vi "HFRR ADV v04 new software.vi"() -> ()   [LabVIEW 2025] (continued)
                n290 = Wait (ms)(milliseconds to wait=u32 1500) -> ()  [unwired: 1 out]
              }
            }
          }
        }
      }
      event "Headen Service Button": Value Change {
        n291 = event-data() -> ()  [unwired: 1 in, 6 out]
        n292 = local read "Headen Service Button"() -> (w388:bool)
        n293 = case shown="True" w388 {
          frame False {
            n294 = property on="Password 3" class="Clust (strict)"("Visible"=FALSE) -> ()  [unwired: 2 in, 2 out]
            n295 = property on="Service Password Log" class="Str"("Visible"=FALSE) -> ()  [unwired: 2 in, 2 out]
          }
          frame True {
            n296 = property on="Password 3" class="Clust (strict)"("Visible"=TRUE) -> ()  [unwired: 2 in, 2 out]
            n297 = property on="Service Password Log" class="Str"("Visible"=TRUE) -> ()  [unwired: 2 in, 2 out]
          }
        }
      }
      event "Password 3.Service Password": Value Change {
        n298 = event-data() -> ()  [unwired: 1 in, 6 out]
        n299 = Unbundle By Name("Password 3") -> ("Service Password"=w395:string)
        n300 = call <vilib>:"Trim Whitespace.vi"("string"=w395) -> ("trimmed string"=w393:string)  [unwired: 1 in]
        n301 = Equal?(x=w393, y="Service@123") -> (x = y?=w394:bool)
        n302 = case shown="False" w394 {
          selector: w394 -> [w399 w401]
          frame False {
            n303 = local write "Service Password enable"(w399) -> ()
            n304 = property on="Service Password Log" class="Str"("Visible"=TRUE) -> ()  [unwired: 2 in, 2 out]
            n305 = property on="Tab Control 5" class="TabCtl (strict)"("Tabs Visible?"=TRUE ("Page Labels Display Visible?")) -> ()  [unwired: 2 in, 2 out]
          }
          frame True {
            n306 = property on="Service Password Log" class="Str"("Visible"=FALSE) -> ()  [unwired: 2 in, 2 out]
            "Service Password enable" <- w401
          }
        }
      }
      event "Sign In": Value Change {
        w403 = FALSE ("Visible")
        n307 = event-data() -> ()  [unwired: 1 in, 6 out]
        n308 = property on="About" class="Clust (strict)"("Visible"=w403) -> ()  [unwired: 2 in, 2 out]
        n309 = property on="Password 3" class="Clust (strict)"("Visible"=w403) -> ()  [unwired: 2 in, 2 out]
        n310 = property on="Service Password Log" class="Str"("Visible"=FALSE) -> ()  [unwired: 2 in, 2 out]
      }
      event "Info": Value Change {
        n311 = event-data() -> ()  [unwired: 1 in, 6 out]
        n312 = local read "Info"() -> (w405:bool)
        n313 = case shown="False" w405 {
          frame False {
            n314 = property on="About" class="Clust (strict)"("Visible"=FALSE) -> ()  [unwired: 2 in, 2 out]
          }
          frame True {
            n315 = property on="About" class="Clust (strict)"("Visible"=TRUE) -> ()  [unwired: 2 in, 2 out]
          }
        }
      }
      event "Calibration": Value Change {
        n316 = event-data() -> ()  [unwired: 1 in, 6 out]
        n317 = local read "Calibration"() -> (w409:bool)
        n318 = case shown="False" w409 {
          frame False {
            n319 = property on="Calibration 2" class="TabCtl (strict)"("Visible"=FALSE) -> ()  [unwired: 2 in, 2 out]
            n320 = local write "Cal Password"("" ("Cal Password")) -> ()
          }
          frame True {
            n321 = property on="Calibration 2" class="TabCtl (strict)"("Visible"=TRUE) -> ()  [unwired: 2 in, 2 out]
            n322 = local write "Cal Password"("" ("Cal Password")) -> ()
          }
        }
        n323 = property on="Wrong Password" class="Str"("Visible"=FALSE) -> ()  [unwired: 2 in, 2 out]
      }
      event "Cal Password": Value Change {
        n324 = event-data() -> ()  [unwired: 1 in, 6 out]
        n325 = local read "Cal Password"() -> (w417:string)
        n326 = call <vilib>:"Trim Whitespace.vi"("string"=w417) -> ("trimmed string"=w416:string)  [unwired: 1 in]
        n327 = Equal?(x=w416, y="Cal@321") -> (x = y?=w414:bool)
        n328 = case shown="True" w414 {
          frame False {
            n329 = property on="Wrong Password" class="Str"("Visible"=TRUE) -> ()  [unwired: 2 in, 2 out]
          }
          frame True {
            n330 = property on="Wrong Password" class="Str"("Visible"=FALSE) -> ()  [unwired: 2 in, 2 out]
            n331 = local write "Main Tab"(T2."About" ("Main Tab")) -> ()
            n332 = local write "Cal Password"("" ("Cal Password")) -> ()
            n333 = local write "Main Dashboard Buttons"(T1."About" ("Main Dashboard Buttons")) -> ()
            n334 = local write "Tab Control 5"(T7."Temperature Calibration" ("Tab Control 5")) -> ()
            n335 = property on="Calibration 2" class="TabCtl (strict)"("Visible"=FALSE) -> ()  [unwired: 2 in, 2 out]
            n336 = property on="Tab Control 5" class="TabCtl (strict)"("Tabs Visible?"=FALSE ("Page Labels Display Visible?")) -> ()  [unwired: 2 in, 2 out]
            n337 = local write "Calibration"(FALSE ("Calibration")) -> ()
          }
        }
      }
      event "Quit": Value Change {
        n338 = event-data() -> ()  [unwired: 1 in, 6 out]
      }
    }
    n339 = Wait (ms)(milliseconds to wait=u32 100) -> ()  [unwired: 1 out]
  }
  n340 = local write "Auto stop temp"(w12) -> ()
  n341 = local write "main tab sub"(enum32{"Page 1", "Page 2"}."Page 1" ("main tab sub")) -> ()
  n342 = local write "USERNAME"(w31) -> ()
  n343 = local write "Main Tab"(T2."HOME" ("Main Tab")) -> ()
  n344 = local write "USER ID"(w31) -> ()
  n345 = property on="Auto Scar Check  2" class="Clust (strict)"("Visible"=w12) -> (error out=w16:errorcluster)  [unwired: 2 in, 1 out]
  n346 = property on="Quit" class="Bool (strict)"("Value"=FALSE ("Quit")) -> (error out=w33:errorcluster)  [unwired: 2 in, 1 out]
  n347 = while {
    shift-right: [w429] -> _
    shift-left: "Enum - Selector" -> [w430]
    stop <- w431 stop-if-true
    # "Auto Start Logic Loop"
    n348 = case shown="\"close\"" w430 {
      tunnel: [w434 w440 w451 w483 w514 Auto_Start_enum."Exit" ("Enum - Selector") Auto_Start_enum."Init" ("Enum - Selector")] -> w429
      frame "Init", Default {
        n349 = local read "Auto Start Test"() -> (w433:bool)
        n350 = Select(t=Auto_Start_enum."Humidity & Temperature On" ("Enum - Selector"), s=w433, f=Auto_Start_enum."Init") -> (s? t:f=w434:T10)
      }
      frame "Humidity & Temperature On" {
        n351 = flat-sequence {
          tunnel: [Auto_Start_enum."Reach point" ("Enum - Selector")] -> w437
          frame #0 {
            w441 = T13."Disabled and Grayed Out" ("Disabled")
            w442 = TRUE ("Heater Button")
            n352 = property on="Humidity" class="Bool (strict)"("DisabledEnum"=w441) -> ()  [unwired: 2 in, 2 out]
            n353 = property on="Heater Button" class="Bool (strict)"("DisabledEnum"=w441) -> ()  [unwired: 2 in, 2 out]
            n354 = local write "Heater Button"(w442) -> ()
            n355 = local write "Humidity"(w442) -> ()
          }
          frame #1 {
            n356 = Wait (ms)(milliseconds to wait=u32 1000) -> ()  [unwired: 1 out]
          }
          frame #2 {
            w444 = TRUE ("Reach point temp")
            n357 = local write "Reach point Humidity"(w444) -> ()
            n358 = local write "Reach point temp"(w444) -> ()
          }
        }
        n359 = local read "Auto Start Test"() -> (w439:bool)
        n360 = Not(x=w439) -> (.not. x?=w438:bool)
        n361 = Select(t=Auto_Start_enum."close", s=w438, f=w437) -> (s? t:f=w440:T10)
      }
      frame "Reach point" {
        w452 = TRUE ("PAUSE")
        w460 = 1.0 ("y")
        w463 = 1.0 ("y")
        n362 = local read "Set Temperature:"() -> (w464:dbl)
        n363 = local read "Set Humidity:"() -> (w459:dbl)
        n364 = local read "Humidity ( %RH )"() -> (w465:dbl)
        n365 = Add(x=w464, y=w463) -> (x+y=w462:dbl)
        n366 = Subtract(x=w464, y=w463) -> (x-y=w461:dbl)
        n367 = Add(x=w459, y=w460) -> (x+y=w458:dbl)
        n368 = Subtract(x=w459, y=w460) -> (x-y=w457:dbl)
        n369 = local read "TEMP"() -> (w466:dbl)
        n370 = In Range and Coerce(upper limit=w458, x=w465, lower limit=w457) -> (In Range?=w446:bool)  [unwired: 1 out]
        n371 = In Range and Coerce(upper limit=w462, x=w466, lower limit=w461) -> (In Range?=w447:bool)  [unwired: 1 out]
        n372 = case shown="True" w446 {
          frame False {
          }
          frame True {
            n373 = case shown="True" "Reach point Humidity" {
              selector: "Reach point Humidity" -> [_ w472]
              frame False {
              }
              frame True {
                n374 = local read "EVENT LOG"() -> (w469:string)
                n375 = Not(x=w472) -> (.not. x?=w471:bool)
                n376 = local write "Reach point Humidity"(w471) -> ()
                n377 = call "Event Log.vi"("Content"="Target Humidity reached", "EVENT LOG"=w469) -> ("EVENT LOG"=w470:string)  [unwired: 8 in, 1 out]
                n378 = local write "EVENT LOG"(w470) -> ()
              }
            }
          }
        }
        n379 = case shown="True" w447 {
          frame False {
          }
          frame True {
            n380 = case shown="True" "Reach point temp" {
              selector: "Reach point temp" -> [_ w478]
              frame False {
              }
              frame True {
                n381 = local read "EVENT LOG"() -> (w475:string)
                n382 = Not(x=w478) -> (.not. x?=w477:bool)
                n383 = local write "Reach point temp"(w477) -> ()
                n384 = call "Event Log.vi"("Content"="Target Temperature reached", "EVENT LOG"=w475) -> ("EVENT LOG"=w476:string)  [unwired: 8 in, 1 out]
                n385 = local write "EVENT LOG"(w476) -> ()
              }
            }
          }
        }
        n386 = local read "Auto Start Test"() -> (w450:bool)
        n387 = And(x=w447, y=w446) -> (x .and. y?=w456:bool)
        n388 = Select(t=Auto_Start_enum."Maintain Stage" ("Enum - Selector"), s=w456, f=Auto_Start_enum."Reach point" ("Enum - Selector")) -> (s? t:f=w453:T10)
        n389 = Not(x=w450) -> (.not. x?=w449:bool)
        n390 = Select(t=Auto_Start_enum."close", s=w449, f=w453) -> (s? t:f=w451:T10)
        n391 = call "ELAPSED TIMER VI.vi"("RESET"=w452, "PAUSE"=w452) -> ()  [unwired: 7 in, 3 out]
      }
      frame "Maintain Stage" {
        w492 = 2.0 ("y")
        w491 = 1.0 ("y")
        # "Humidity and  temperatures Set Point  have been reached"
        n392 = local read "Set Temperature:"() -> (w498:dbl)
        n393 = local read "Set Humidity:"() -> (w495:dbl)
        n394 = local read "Humidity ( %RH )"() -> (w499:dbl)
        n395 = Add(x=w498, y=w491) -> (x+y=w497:dbl)
        n396 = Subtract(x=w498, y=w491) -> (x-y=w496:dbl)
        n397 = local read "TEMP"() -> (w500:dbl)
        n398 = Add(x=w495, y=w492) -> (x+y=w494:dbl)
        n399 = Subtract(x=w495, y=w492) -> (x-y=w493:dbl)
        n400 = In Range and Coerce(upper limit=w497, x=w500, lower limit=w496) -> (In Range?=w490:bool)  [unwired: 1 out]
        n401 = In Range and Coerce(upper limit=w494, x=w499, lower limit=w493) -> (In Range?=w489:bool)  [unwired: 1 out]
        n402 = And(x=w490, y=w489) -> (x .and. y?=w488:bool)
        n403 = Not(x=w488) -> (.not. x?=w487:bool)
        n404 = call "ELAPSED TIMER VI.vi"("TARGET"=60.0, "RESET"=w487, "PAUSE"=FALSE) -> ("ELAPSED INDICATION"=w484:bool)  [unwired: 6 in, 2 out]
        n405 = case shown="True" w484 {
          tunnel: w484 -> [_ w503]
          tunnel: [Auto_Start_enum."Maintain Stage" ("Enum - Selector") w502] -> w482
          frame False {
          }
          frame True {
            n406 = stacked-sequence {
              tunnel: w503 -> [_ _ _ _ _]
              tunnel: [_ _ _ _ Auto_Start_enum."Start Stage" ("Enum - Selector")] -> w502
              frame #0 {
                n407 = local read "EVENT LOG"() -> (w505:string)
                n408 = call "Event Log.vi"("Content"="Humidity and temperature set point has stabilized.", "EVENT LOG"=w505) -> ("EVENT LOG"=w506:string)  [unwired: 8 in, 1 out]
                n409 = local write "EVENT LOG"(w506) -> ()
              }
              frame #1 {
                n410 = Wait (ms)(milliseconds to wait=u32 100) -> ()  [unwired: 1 out]
              }
              frame #2 {
                n411 = local read "EVENT LOG"() -> (w509:string)
                n412 = call "Event Log.vi"("Content"="Auto Test Started", "EVENT LOG"=w509) -> ("EVENT LOG"=w510:string)  [unwired: 8 in, 1 out]
                n413 = local write "EVENT LOG"(w510) -> ()
              }
              frame #3 {
                w511 = TRUE ("RUN")
                n414 = local write "RUN"(w511) -> ()
                "Auto Start Temp" <- w511
              }
              frame #4 {
              }
            }
          }
        }
        n415 = local read "Auto Start Test"() -> (w481:bool)
        n416 = Not(x=w481) -> (.not. x?=w480:bool)
        n417 = Select(t=Auto_Start_enum."close", s=w480, f=w482) -> (s? t:f=w483:T10)
      }
      frame "Start Stage" {
        w513 = TRUE ("PAUSE")
        n418 = local read "Auto Start Test"() -> (w518:bool)
        n419 = Not(x=w518) -> (.not. x?=w517:bool)
        n420 = Select(t=Auto_Start_enum."close" ("Enum - Selector"), s=w517, f=Auto_Start_enum."Start Stage" ("Enum - Selector")) -> (s? t:f=w514:T10)
        n421 = call "ELAPSED TIMER VI.vi"("RESET"=w513, "PAUSE"=w513) -> ()  [unwired: 7 in, 3 out]
      }
      frame "close" {
        w519 = FALSE ("Heater Button")
        n422 = local write "RUN"(w519) -> ()
        n423 = local write "Heater Button"(w519) -> ()
        n424 = local write "Humidity"(w519) -> ()
        n425 = local write "Auto Start Test"(w519) -> ()
      }
      frame "Exit" {
      }
    }
    n426 = Wait (ms)(milliseconds to wait=u32 100) -> ()  [unwired: 1 out]
    n427 = local read "Quit"() -> (w431:bool)
  }
  n428 = while {
    stop <- w548 stop-if-true
    w531 = errorcluster {"status"=FALSE, "code"=0, "source"=""} ("error in (no error) 3")
    # "this loop is for manual report generation"
    n429 = local read "Confirm Measrurement"() -> (w530:bool)
    n430 = case shown="True" w530 {
      selector: w530 -> [_ w638]
      tunnel: errorcluster {"status"=FALSE, "code"=0, "source"=""} ("error in (no error) 3") -> [_ w639]
      tunnel: [_ w637] -> _
      frame False {
      }
      frame True {
        n431 = stacked-sequence {
          tunnel: w639 -> [_ w672 _]
          tunnel: w638 -> [_ _ w779]
          tunnel: [_ w660 _] -> w637
          frame #0 {
            n432 = String To Path(string="C:\\LAB-IQ\\Image Calibrate v01.dcf") -> (path=w642:path)
            n433 = Open/Create/Replace File ("Open File")(file path (use dialog)=w642) -> (refnum out=w643:refnum<file>)  [unwired: 5 in, 2 out]
            n434 = for {
              N: 4 -> [_]
              tunnel: w643 -> [w649]
              i -> [w645]
              n435 = Read from Text File ("Read File")(file (use dialog)=w649) -> (text=w650:string)  [unwired: 3 in, 3 out]
              n436 = String Subset(string=w650, offset (0)=6, length (rest)=10 ("length (rest)")) -> (substring=w646:string)
              n437 = Fract/Exp String To Number(string=w646) -> (number=w644:dbl)  [unwired: 3 in, 1 out]
              n438 = case shown="3" w645 {
                tunnel: w644 -> [w651 w652 _ w653 _]
                frame 0 {
                  n439 = local write "5x Gain"(w651) -> ()
                }
                frame 1 {
                  n440 = local write "10x Gain"(w652) -> ()
                }
                frame 2 {
                }
                frame 3 {
                  n441 = local write "100x gain"(w653) -> ()
                }
                frame 4, Default {
                }
              }
            }
          }
          frame #1 {
            n442 = local read "TEST STANDARD"() -> (w655:T3)
            n443 = case shown="\"ISO 12156\"" w655 {
              tunnel: ["ASTM D6079" "ISO 12156"] -> w654
              frame "ASTM D6079", Default {
              }
              frame "ISO 12156" {
              }
            }
            n444 = call "IMAGE ANALYSIS.vi"("Enum"=POST_ANALYSIS_ENUM."GET MEASUREMENTS", "error in"=w672) -> ("error out"=w679:errorcluster)  [unwired: 8 in, 1 out]
            n445 = local read "Magnification :"() -> (w665:string)
            n446 = call "Stall Data Flow.vim"("value in"=w679, "milliseconds to wait"=u32 1000) -> ("value out"=w678:errorcluster)  [unwired: 1 out]
            n447 = local read "Test File List :"() -> (w676:string)
            n448 = case shown="\"10x\"" w665 {
              tunnel: [w715 w716] -> w663
              frame "5x", Default {
                n449 = local read "5x Gain"() -> (w715:dbl)
              }
              frame "10x" {
                # "5x"
                n450 = local read "10x Gain"() -> (w716:dbl)
              }
            }
            n451 = call "IMAGE ANALYSIS.vi"("Enum"=POST_ANALYSIS_ENUM."READ", "error in"=w678) -> ("error out"=w675:errorcluster, "data out"=w666:string)  [unwired: 8 in]
            n452 = Match Pattern(string=w666, regular expression="\"type\": ") -> (after substring=w670:string)  [unwired: 1 in, 3 out]
            n453 = call "IMAGE PATH CREATION PY.vi"("error in (no error)"=w675, "File Name :"=w676) -> ("error out"=w674:errorcluster, "File Path"=w662:path, "File Path String:"=w657:string)  [unwired: 7 in]
            n454 = Match Pattern(string=w670, regular expression=",") -> (before substring=w656:string)  [unwired: 1 in, 3 out]
            n455 = local read "Calibration Tab"() -> (w659:enum32{"Measrument", "Calibrate"})
            n456 = call "Stall Data Flow.vim"("value in"=w674, "milliseconds to wait"=u32 250) -> ("value out"=w658:errorcluster)  [unwired: 1 out]
            n457 = Equal?(x=w656, y="\"rectangle\"") -> (x = y?=w667:bool)
            n458 = case shown="False" w667 {
              tunnel: w666 -> [w721 w776]
              tunnel: w663 -> [_ w767]
              tunnel: cluster{"major":dbl, "minor":dbl, "average":dbl} {"major"=0.0, "minor"=0.0, "average"=0.0} -> [w719 w763]
              tunnel: [w718 w760] -> w661
              tunnel: w656 -> [w720 _]
              tunnel: w663 -> [w717 _]
              frame False {
                n459 = Equal?(x=w720, y="\"line\"") -> (x = y?=w722:bool)
                n460 = case shown="True" w722 {
                  tunnel: w721 -> [_ w737]
                  tunnel: w719 -> [w724 w736]
                  tunnel: [w724 w734] -> w718
                  tunnel: w717 -> [_ w733]
                  frame False {
                  }
                  frame True {
                    w732 = 0.0 ("Major Axis")
                    n461 = Match Pattern(string=w737, regular expression="\"length_px\":") -> (after substring=w735:string)  [unwired: 1 in, 3 out]
                    n462 = property on="Major Axis" class="DigNum (strict)"("Caption.Text"="") -> ()  [unwired: 2 in, 2 out]
                    n463 = property on="Minor Axis" class="DigNum (strict)"("Caption.Text"="") -> ()  [unwired: 2 in, 2 out]
                    n464 = property on="Average" class="DigNum (strict)"("Caption.Text"="Line") -> ()  [unwired: 2 in, 2 out]
                    n465 = Fract/Exp String To Number(string=w735, default (0 dbl)=0.0 ("default (0 DBL)")) -> (number=w731:dbl)  [unwired: 2 in, 1 out]
                    "Pixel Value" <- w731
                    n466 = Multiply(x=w731, y=w733) -> (x*y=w744:dbl)
                    n467 = Multiply(x=w744, y=1000.0) -> (x*y=w727:dbl)
                    n468 = Divide(x=w727, y=1000.0) -> (x/y=w730:dbl)
                    n469 = local write "Measurment (mm)"(w730) -> ()
                    n470 = Bundle By Name(cluster=w736, "average"=w727) -> (w734:cluster{"major":dbl, "minor":dbl, "average":dbl})
                    n471 = Number To Fractional String(number=w727, precision (6)=i16 1) -> (F-format string=w726:string)  [unwired: 2 in]
                    n472 = local write "Minor Axis"(w732) -> ()
                    n473 = local write "Major Axis"(w732) -> ()
                    n474 = Fract/Exp String To Number(string=w726) -> (number=w725:dbl)  [unwired: 3 in, 1 out]
                    n475 = local write "Average"(w725) -> ()
                  }
                }
              }
              frame True {
                w764 = 1000.0 ("y")
                w770 = 0.0 ("default (0 DBL)")
                n476 = Match Pattern(string=w776, regular expression=" \"width_px\":") -> (after substring=w774:string)  [unwired: 1 in, 3 out]
                n477 = Match Pattern(string=w774, regular expression="\"height_px\":") -> (before substring=w772:string, after substring=w771:string)  [unwired: 1 in, 2 out]
                n478 = Fract/Exp String To Number(string=w772, default (0 dbl)=w770) -> (number=w769:dbl)  [unwired: 2 in, 1 out]
                n479 = Fract/Exp String To Number(string=w771, default (0 dbl)=w770) -> (number=w768:dbl)  [unwired: 2 in, 1 out]
                n480 = Multiply(x=w769, y=w767) -> (x*y=w766:dbl)
                n481 = Multiply(x=w768, y=w767) -> (x*y=w765:dbl)
                n482 = Multiply(x=w766, y=w764) -> (x*y=w750:dbl)
                n483 = Multiply(x=w765, y=w764) -> (x*y=w748:dbl)
                n484 = Add(x=w750, y=w748) -> (x+y=w762:dbl)
                n485 = property on="Major Axis" class="DigNum (strict)"("Caption.Text"="Major Axis") -> ()  [unwired: 2 in, 2 out]
                n486 = property on="Minor Axis" class="DigNum (strict)"("Caption.Text"="Minor Axis") -> ()  [unwired: 2 in, 2 out]
                n487 = property on="Average" class="DigNum (strict)"("Caption.Text"="Average") -> ()  [unwired: 2 in, 2 out]
                n488 = Divide(x=w762, y=2.0) -> (x/y=w746:dbl)
                n489 = Bundle By Name(cluster=w763, "major"=w750, "minor"=w748, "average"=w746) -> (w760:cluster{"major":dbl, "minor":dbl, "average":dbl})
                n490 = Number To Fractional String(number=w748, precision (6)=i16 1) -> (F-format string=w755:string)  [unwired: 2 in]
                n491 = Number To Fractional String(number=w746, precision (6)=i16 1) -> (F-format string=w756:string)  [unwired: 2 in]
                n492 = Number To Fractional String(number=w750, precision (6)=i16 1) -> (F-format string=w754:string)  [unwired: 2 in]
                n493 = Fract/Exp String To Number(string=w755) -> (number=w747:dbl)  [unwired: 3 in, 1 out]
                n494 = Fract/Exp String To Number(string=w756) -> (number=w745:dbl)  [unwired: 3 in, 1 out]
                n495 = Fract/Exp String To Number(string=w754) -> (number=w749:dbl)  [unwired: 3 in, 1 out]
                n496 = local write "Major Axis"(w749) -> ()
                n497 = local write "Average"(w745) -> ()
                n498 = local write "Minor Axis"(w747) -> ()
              }
            }
            n499 = case shown="\"Measrument\", Default" w659 {
              tunnel: w662 -> [w689 _]
              tunnel: w661 -> [w688 _]
              tunnel: [w685 w714] -> w660
              tunnel: w658 -> [w687 w714]
              tunnel: w657 -> [w686 _]
              tunnel: w654 -> [w684 _]
              frame "Measrument", Default {
                n500 = stacked-sequence {
                  tunnel: w689 -> [w707 _]
                  tunnel: w688 -> [w705 _]
                  tunnel: w687 -> [w703 _]
                  tunnel: w686 -> [w702 _]
                  tunnel: [w697 _] -> w685
                  tunnel: w684 -> [w690 _]
                  frame #0 {
                    n501 = call "IMAGE ANALYSIS.vi"("Enum"=POST_ANALYSIS_ENUM."SAVE IMAGE", "error in"=w703, "IMAGE FILE PATH"=w702) -> ("error out"=w701:errorcluster)  [unwired: 7 in, 1 out]
                    n502 = call "Stall Data Flow.vim"("value in"=w701, "milliseconds to wait"=u32 1000) -> ("value out"=w692:errorcluster)  [unwired: 1 out]
                    n503 = local read "Test File List :"() -> (w709:string)
                    n504 = call "IMAGE ANALYSIS.vi"("Enum"=POST_ANALYSIS_ENUM."MINIMIZE UI", "error in"=w692) -> ("error out"=w699:errorcluster)  [unwired: 8 in, 1 out]
                    n505 = Bundle By Name(cluster=T18 {"File Name"="", "Test Method"="", "Operator"="", "Fuel Description"="", "Date and time"=""} ("Main Ref"), "Test Method"=w690, "File Name"=w709) -> (w710:T18)
                    n506 = call "Stall Data Flow.vim"("value in"=w699, "milliseconds to wait"=u32 1500) -> ("value out"=w694:errorcluster)  [unwired: 1 out]
                    n507 = call "duf file read.vi"("error in (no error)"=w694, "Main Ref"=w710) -> ("error out"=w708:errorcluster, "Main Ref 2"=w706:T18)  [unwired: 8 in]
                    n508 = call "DETECTION REPORT for manual.vi"("error in (no error)"=w708, "return value 3"=w705, "Image File Path"=w707, "Main Ref"=w706) -> ("error out"=w704:errorcluster)  [unwired: 7 in]
                    n509 = call <vilib>:"Clear Errors.vi"("error in (no error)"=w704) -> ("error out"=w695:errorcluster)  [unwired: 5 in, 1 out]
                    n510 = call "IMAGE ANALYSIS.vi"("Enum"=POST_ANALYSIS_ENUM."MINIMIZE UI", "error in"=w695) -> ("error out"=w697:errorcluster)  [unwired: 8 in, 1 out]
                  }
                  frame #1 {
                    n511 = local write "Main Tab"(T2."HOME" ("Main Tab")) -> ()
                    n512 = local write "Main Dashboard Buttons"(T1."Home" ("Main Dashboard Buttons")) -> ()
                  }
                }
              }
              frame "Calibrate" {
              }
            }
          }
          frame #2 {
            n513 = Not(x=w779) -> (.not. x?=w778:bool)
            n514 = local write "Confirm Measrurement"(w778) -> ()
            n515 = local read "Calibration Tab"() -> (w777:enum32{"Measrument", "Calibrate"})
            n516 = case shown="\"Measrument\", Default" w777 {
              frame "Measrument", Default {
                n517 = local write "Main Tab"(T2."HOME" ("Main Tab")) -> ()
              }
              frame "Calibrate" {
              }
            }
          }
        }
      }
    }
    n518 = local read "Humidity"() -> (w522:bool)
    n519 = local read "Save Change"() -> (w527:bool)
    n520 = local read "Calibrate"() -> (w528:bool)
    n521 = local read "Auto Start Test"() -> (w523:bool)
    n522 = case shown="True" w528 {
      selector: w528 -> [_ w635]
      frame False {
      }
      frame True {
        n523 = Not(x=w635) -> (.not. x?=w634:bool)
        n524 = local write "Calibrate"(w634) -> ()
        n525 = local write "Calibration Tab"(enum32{"Measrument", "Calibrate"}."Calibrate" ("Calibration Tab")) -> ()
      }
    }
    n526 = case shown="True" w527 {
      selector: w527 -> [_ w579]
      frame False {
      }
      frame True {
        n527 = stacked-sequence {
          tunnel: w579 -> [_ _ _ _ w633]
          frame #0 {
            n528 = call "IMAGE ANALYSIS.vi"("Enum"=POST_ANALYSIS_ENUM."HIDE UI") -> ()  [unwired: 9 in, 2 out]
          }
          frame #1 {
            n529 = local read "100x gain"() -> (w581:dbl)
            n530 = local read "10x Gain"() -> (w582:dbl)
            n531 = local read "5x Gain"() -> (w583:dbl)
            n532 = Number To Fractional String(number=w582, width (-)=i16 4, precision (6)=i16 7) -> (F-format string=w604:string)  [unwired: 1 in]
            n533 = Number To Fractional String(number=0.0, width (-)=i16 4, precision (6)=i16 7) -> (F-format string=w599:string)  [unwired: 1 in]
            n534 = Number To Fractional String(number=w581, width (-)=i16 4, precision (6)=i16 7) -> (F-format string=w587:string)  [unwired: 1 in]
            n535 = Number To Fractional String(number=w583, width (-)=i16 10 ("precision (6)"), precision (6)=i16 7) -> (F-format string=w613:string)  [unwired: 1 in]
            n536 = Concatenate Strings("[CH1]" ("string"), w613, " - 5x Gain" ("string"), "\r") -> (w603:string)
            n537 = Concatenate Strings("[CH2]" ("string"), w604, " - 10x Gain" ("string"), "\r") -> (w602:string)
            n538 = Concatenate Strings("[CH3]" ("string"), w599, " - 20x Gain" ("string"), "\r") -> (w593:string)
            n539 = Concatenate Strings("[CH4]" ("string"), w587, " - 100x Gain" ("string"), "\r") -> (w586:string)
            n540 = String To Path(string="C:\\LAB-IQ\\Image Calibrate v01.dcf") -> (path=w616:path)
            n541 = Concatenate Strings(w603, w602, w593, w586) -> (w601:string)
            n542 = call <vilib>:"Write Characters To File.vi"("append to file? (new file:F)"=FALSE, "character string"=w601, "file path (dialog if empty)"=w616) -> ()  [unwired: 2 in, 1 out]
          }
          frame #2 {
            n543 = String To Path(string="C:\\LAB-IQ\\Image Calibrate v01.dcf") -> (path=w619:path)
            n544 = Open/Create/Replace File ("Open File")(file path (use dialog)=w619) -> (refnum out=w620:refnum<file>)  [unwired: 5 in, 2 out]
            n545 = for {
              N: 4 -> [_]
              tunnel: w620 -> [w626]
              i -> [w622]
              n546 = Read from Text File ("Read File")(file (use dialog)=w626) -> (text=w627:string)  [unwired: 3 in, 3 out]
              n547 = String Subset(string=w627, offset (0)=6, length (rest)=10 ("length (rest)")) -> (substring=w623:string)
              n548 = Fract/Exp String To Number(string=w623) -> (number=w621:dbl)  [unwired: 3 in, 1 out]
              n549 = case shown="3" w622 {
                tunnel: w621 -> [w628 w629 _ w630 _]
                frame 0 {
                  n550 = local write "5x Gain"(w628) -> ()
                }
                frame 1 {
                  n551 = local write "10x Gain"(w629) -> ()
                }
                frame 2 {
                }
                frame 3 {
                  n552 = local write "100x gain"(w630) -> ()
                }
                frame 4, Default {
                }
              }
            }
          }
          frame #3 {
            n553 = call "IMAGE ANALYSIS.vi"("Enum"=POST_ANALYSIS_ENUM."SHOW UI") -> ()  [unwired: 9 in, 2 out]
          }
          frame #4 {
            n554 = Not(x=w633) -> (.not. x?=w632:bool)
            n555 = local write "Save Change"(w632) -> ()
          }
        }
      }
    }
    n556 = case shown="False" w523 {
      tunnel: w522 -> [w549 _]
      frame False {
        n557 = case shown="True" w549 {
          frame False {
          }
          frame True {
            n558 = local read "Set Humidity:"() -> (w553:dbl)
            n559 = local read "Set Humidity:"() -> (w556:dbl)
            n560 = local read "Humidity ( %RH )"() -> (w557:dbl)
            n561 = Subtract(x=w553, y=2.0) -> (x-y=w551:dbl)
            n562 = Add(x=w556, y=2.0) -> (x+y=w552:dbl)
            n563 = In Range and Coerce(upper limit=w552, x=w557, lower limit=w551) -> (In Range?=w550:bool)  [unwired: 1 out]
            n564 = case shown="True" w550 {
              frame False {
              }
              frame True {
                n565 = case shown="False" "Manual Humididty Reached" {
                  selector: "Manual Humididty Reached" -> [_ w560]
                  frame False {
                  }
                  frame True {
                    n566 = Not(x=w560) -> (.not. x?=w559:bool)
                    n567 = local write "Manual Humididty Reached"(w559) -> ()
                    n568 = local read "EVENT LOG"() -> (w562:string)
                    n569 = call "Event Log.vi"("Content"="Target Humidity reached", "EVENT LOG"=w562) -> ("EVENT LOG"=w561:string)  [unwired: 8 in, 1 out]
                    n570 = local write "EVENT LOG"(w561) -> ()
                  }
                }
              }
            }
          }
        }
      }
      frame True {
        n571 = local write "Manual Humididty Reached"(TRUE ("Manual Humididty Reached")) -> ()
      }
    }
    n572 = local read "Cap Live Image"() -> (w543:bool)
    n573 = local read "SCAR MEASURMENT"() -> (w546:enum32{"Auto Scar", "Manual Scar"})
    n574 = Wait (ms)(milliseconds to wait=u32 250) -> ()  [unwired: 1 out]
    n575 = Equal?(x=w546, y=enum32{"Auto Scar", "Manual Scar"}."Manual Scar" ("SCAR MEASURMENT")) -> (x = y?=w544:bool)
    n576 = And(x=w544, y=w543) -> (x .and. y?=w542:bool)
    n577 = case shown="True" w542 {
      selector: w542 -> [_ w858]
      frame False {
      }
      frame True {
        n578 = stacked-sequence {
          tunnel: [_ _ _ w873 _] -> _
          tunnel: w858 -> [_ _ _ _ w879]
          frame #0 {
            w859 = 0.0
            n579 = local write "Major Axis"(w859) -> ()
            n580 = local write "Minor Axis"(w859) -> ()
            n581 = local write "Average"(w859) -> ()
          }
          frame #1 {
            n582 = call "CAMERA LIVE FEED FGV.vi"("Enum - Menu"=CAMERA_LIVE_FEED_ENUM."CAMERA MINIMIZE") -> ()  [unwired: 9 in, 2 out]
          }
          frame #2 {
            n583 = local read "FILE 3"() -> (w867:string)
            n584 = call <vilib>:"Trim Whitespace.vi"("string"="C:\\LAB-IQ\\images\\") -> ("trimmed string"=w869:string)  [unwired: 1 in]
            n585 = String To Path(string=w869) -> (path=w868:path)
            n586 = Concatenate Strings(w867, ".png" ("string")) -> (w866:string)
            n587 = Build Path(base path=w868, name or relative path=w866) -> (appended path=w864:path)
            n588 = Path To String(path=w864) -> (string=w863:string)
            n589 = call "CAMERA LIVE FEED FGV.vi"("Enum - Menu"=CAMERA_LIVE_FEED_ENUM."CAMERA SAVE", "Image Path"=w863) -> ("error out"=w861:errorcluster)  [unwired: 8 in, 1 out]
            n590 = case shown="No Error" w861 {
              frame No Error {
                n591 = One Button Dialog(message="Image saved successfully") -> ()  [unwired: 1 in, 1 out]
              }
              frame Error {
              }
            }
          }
          frame #3 {
            n592 = call "LIST FILE NAMES.vi"() -> ("error out"=w875:errorcluster, "filenames"=w872:string[])  [unwired: 10 in]
            n593 = call "IMAGE ANALYSIS.vi"("Enum"=POST_ANALYSIS_ENUM."SHOW UI", "error in"=w875) -> ("error out"=w873:errorcluster)  [unwired: 8 in, 1 out]
            n594 = property on="Test File List :" class="CmbBox"("Strings[]"=w872) -> ()  [unwired: 2 in, 2 out]
          }
          frame #4 {
            (unwired) T19."Report" ("Main Dashboard Buttons")
            n595 = Not(x=w879) -> (.not. x?=w878:bool)
            n596 = local write "Zoom Factore"(0.0 ("Zoom Factore")) -> ()
            n597 = local write "Cap Live Image"(w878) -> ()
            n598 = local write "Main Tab"(T2."Adv Scar Report" ("Main Tab")) -> ()
            n599 = property on="Cap Live Image" class="Bool (strict)"("BoolText.Text"="Capture Image" ("Boolean Text.Text")) -> ()  [unwired: 2 in, 2 out]
            n600 = local write "Main Dashboard Buttons"(T1."Report" ("Main Dashboard Buttons")) -> ()
          }
        }
      }
    }
    n601 = local read "change Gain"() -> (w526:bool)
    n602 = local read "Back Square"() -> (w525:bool)
    n603 = case shown="True" w526 {
      selector: w526 -> [_ w570]
      frame False {
      }
      frame True {
        n604 = stacked-sequence {
          tunnel: w570 -> [_ w578]
          frame #0 {
            n605 = local read "Actual (µm)"() -> (w574:dbl)
            n606 = local read "Pixel Value"() -> (w573:dbl)
            n607 = local read "Magnification :"() -> (w572:string)
            n608 = Divide(x=w574, y=w573) -> (x/y=w571:dbl)
            n609 = case shown="\"10x\"" w572 {
              tunnel: w571 -> [w575 w576]
              frame "10x" {
                n610 = local write "10x Gain"(w575) -> ()
              }
              frame "5x", Default {
                n611 = local write "5x Gain"(w576) -> ()
              }
            }
          }
          frame #1 {
            n612 = Not(x=w578) -> (.not. x?=w577:bool)
            n613 = local write "change Gain"(w577) -> ()
          }
        }
      }
    }
    n614 = case shown="True" w525 {
      selector: w525 -> [_ w568]
      frame False {
      }
      frame True {
        n615 = Not(x=w568) -> (.not. x?=w567:bool)
        n616 = local write "Back Square"(w567) -> ()
        n617 = local write "Calibration Tab"(enum32{"Measrument", "Calibrate"}."Measrument" ("Calibration Tab")) -> ()
      }
    }
    n618 = local read "Rectangle Tool"() -> (w537:bool)
    n619 = local read "Clear ROI Tool"() -> (w536:bool)
    n620 = local read "Open Image"() -> (w541:bool)
    n621 = local read "line tool"() -> (w538:bool)
    n622 = local read "OUT"() -> (w539:bool)
    n623 = local read "In"() -> (w540:bool)
    n624 = case shown="True" w541 {
      selector: w541 -> [_ w846]
      tunnel: [w842 w848] -> _
      tunnel: w531 -> [w842 w847]
      frame False {
      }
      frame True {
        n625 = Not(x=w846) -> (.not. x?=w845:bool)
        n626 = local write "Open Image"(w845) -> ()
        n627 = call "IMAGE ANALYSIS.vi"("Enum"=POST_ANALYSIS_ENUM."HIDE UI", "error in"=w847) -> ("error out"=w855:errorcluster)  [unwired: 8 in, 1 out]
        n628 = call "File Dialog"("start path"=path "C:/LAB-IQ/images", "error in"=w855) -> ("selected path"=w844:path, "error out"=w853:errorcluster)  [unwired: 10 in, 2 out]
        "Image path  2" <- w844
        n629 = call <vilib>:"Clear Errors.vi"("error in (no error)"=w853) -> ("error out"=w852:errorcluster)  [unwired: 5 in, 1 out]
        n630 = call "IMAGE ANALYSIS.vi"("Enum"=POST_ANALYSIS_ENUM."OPEN FILE", "error in"=w852, "File Path"=w844) -> ("error out"=w851:errorcluster)  [unwired: 7 in, 1 out]
        n631 = call <vilib>:"Clear Errors.vi"("error in (no error)"=w851) -> ("error out"=w850:errorcluster)  [unwired: 5 in, 1 out]
        n632 = call "IMAGE ANALYSIS.vi"("Enum"=POST_ANALYSIS_ENUM."SHOW UI", "error in"=w850) -> ("error out"=w848:errorcluster)  [unwired: 8 in, 1 out]
        n633 = local write "Zoom Factore"(100.0 ("Zoom Factore")) -> ()
      }
    }
    n634 = case shown="True" w539 {
      selector: w539 -> [_ w827]
      tunnel: w531 -> [w824 w832]
      tunnel: [w824 w826] -> _
      frame False {
      }
      frame True {
        n635 = Not(x=w827) -> (.not. x?=w825:bool)
        n636 = local read "Zoom Factore"() -> (w830:dbl)
        n637 = local write "OUT"(w825) -> ()
        n638 = call "IMAGE ANALYSIS.vi"("Enum"=POST_ANALYSIS_ENUM."ZOOM OUT", "error in"=w832) -> ("error out"=w826:errorcluster)  [unwired: 8 in, 1 out]
        n639 = Divide(x=w830, y=1.2) -> (x/y=w828:dbl)
        n640 = local write "Zoom Factore"(w828) -> ()
      }
    }
    n641 = case shown="True" w540 {
      selector: w540 -> [_ w836]
      tunnel: w531 -> [w833 w841]
      tunnel: [w833 w834] -> _
      frame False {
      }
      frame True {
        n642 = Not(x=w836) -> (.not. x?=w835:bool)
        n643 = local read "Zoom Factore"() -> (w839:dbl)
        n644 = local write "In"(w835) -> ()
        n645 = call "IMAGE ANALYSIS.vi"("Enum"=POST_ANALYSIS_ENUM."ZOOM IN", "error in"=w841) -> ("error out"=w834:errorcluster)  [unwired: 8 in, 1 out]
        n646 = Multiply(x=w839, y=1.2) -> (x*y=w837:dbl)
        n647 = local write "Zoom Factore"(w837) -> ()
      }
    }
    n648 = case shown="True" w536 {
      selector: w536 -> [_ w808]
      tunnel: w531 -> [w806 w810]
      tunnel: [w806 w809] -> _
      frame False {
      }
      frame True {
        n649 = Not(x=w808) -> (.not. x?=w807:bool)
        n650 = local write "Clear ROI Tool"(w807) -> ()
        n651 = call "IMAGE ANALYSIS.vi"("Enum"=POST_ANALYSIS_ENUM."CLEAR ROI", "error in"=w810) -> ("error out"=w809:errorcluster)  [unwired: 8 in, 1 out]
      }
    }
    n652 = case shown="True" w538 {
      selector: w538 -> [_ w820]
      tunnel: w531 -> [w818 w823]
      tunnel: [w818 w821] -> _
      frame False {
      }
      frame True {
        n653 = Not(x=w820) -> (.not. x?=w819:bool)
        n654 = local write "line tool"(w819) -> ()
        n655 = call "IMAGE ANALYSIS.vi"("Enum"=POST_ANALYSIS_ENUM."DRAW LINE", "error in"=w823) -> ("error out"=w821:errorcluster)  [unwired: 8 in, 1 out]
      }
    }
    n656 = case shown="True" w537 {
      selector: w537 -> [_ w814]
      tunnel: w531 -> [w812 w816]
      tunnel: [w812 w815] -> _
      frame False {
      }
      frame True {
        n657 = Not(x=w814) -> (.not. x?=w813:bool)
        n658 = local write "Rectangle Tool"(w813) -> ()
        n659 = call "IMAGE ANALYSIS.vi"("Enum"=POST_ANALYSIS_ENUM."DRAW REC", "error in"=w816) -> ("error out"=w815:errorcluster)  [unwired: 8 in, 1 out]
      }
    }
    n660 = local read "SCAR MEASURMENT"() -> (w524:enum32{"Auto Scar", "Manual Scar"})
    n661 = local read "Fit to Screen Tool"() -> (w533:bool)
    n662 = local read "Resize Tool"() -> (w532:bool)
    n663 = case shown="\"Manual Scar\", Default" w524 {
      frame "Auto Scar" {
        n664 = property on="Cap Live Image" class="Bool (strict)"("BoolText.Text"="Report" ("Boolean Text.Text")) -> ()  [unwired: 2 in, 2 out]
      }
      frame "Manual Scar", Default {
        n665 = property on="Cap Live Image" class="Bool (strict)"("BoolText.Text"="Save Image" ("Boolean Text.Text")) -> ()  [unwired: 2 in, 2 out]
      }
    }
    n666 = local read "ROI Color Tool"() -> (w534:bool)
    n667 = local read "Pan Tool"() -> (w535:bool)
    n668 = case shown="True" w535 {
      selector: w535 -> [_ w802]
      tunnel: w531 -> [w800 w804]
      tunnel: [w800 w803] -> _
      frame False {
      }
      frame True {
        n669 = Not(x=w802) -> (.not. x?=w801:bool)
        n670 = call "IMAGE ANALYSIS.vi"("Enum"=POST_ANALYSIS_ENUM."PAN", "error in"=w804) -> ("error out"=w803:errorcluster)  [unwired: 8 in, 1 out]
        n671 = local write "Pan Tool"(w801) -> ()
      }
    }
    n672 = case shown="True" w532 {
      selector: w532 -> [_ w786]
      tunnel: w531 -> [w781 w783]
      tunnel: [w781 w782] -> _
      frame False {
      }
      frame True {
        n673 = Not(x=w786) -> (.not. x?=w785:bool)
        n674 = local write "Resize Tool"(w785) -> ()
        n675 = call "IMAGE ANALYSIS.vi"("Enum"=POST_ANALYSIS_ENUM."RESIZE MODE", "error in"=w783) -> ("error out"=w782:errorcluster)  [unwired: 8 in, 1 out]
      }
    }
    n676 = case shown="True" w533 {
      selector: w533 -> [_ w791]
      tunnel: [w787 w792] -> _
      tunnel: w531 -> [w787 w790]
      frame False {
      }
      frame True {
        n677 = Not(x=w791) -> (.not. x?=w789:bool)
        n678 = local write "Zoom Factore"(100.0 ("Zoom Factore")) -> ()
        n679 = local write "Fit to Screen Tool"(w789) -> ()
        n680 = call "IMAGE ANALYSIS.vi"("Enum"=POST_ANALYSIS_ENUM."FIT", "error in"=w790) -> ("error out"=w792:errorcluster)  [unwired: 8 in, 1 out]
      }
    }
    n681 = case shown="True" w534 {
      selector: w534 -> [_ w797]
      tunnel: [w794 w798] -> _
      tunnel: w531 -> [w794 w795]
      frame False {
      }
      frame True {
        n682 = Not(x=w797) -> (.not. x?=w796:bool)
        n683 = local write "ROI Color Tool"(w796) -> ()
        n684 = call "IMAGE ANALYSIS.vi"("Enum"=POST_ANALYSIS_ENUM."SET ROI COLOR", "error in"=w795) -> ("error out"=w798:errorcluster)  [unwired: 8 in, 1 out]
      }
    }
    n685 = local read "Quit"() -> (w548:bool)
  }
  n686 = property on="Service Password Log" class="Str"("Visible"=w12) -> ()  [unwired: 2 in, 2 out]
  n687 = property on="Password 3" class="Clust (strict)"("Visible"=w12) -> ()  [unwired: 2 in, 2 out]
  n688 = while {
    stop <- w882 stop-if-true
    n689 = local read "Image Path"() -> (w885:path)
    n690 = local read "Print 3"() -> (w888:bool)
    n691 = Equal?(x=w885, y=path "") -> (x = y?=w884:bool)
    n692 = Not(x=w884) -> (.not. x?=w883:bool)
    n693 = property on="Print 3" class="Bool (strict)"("Visible"=w883) -> ()  [unwired: 2 in, 2 out]
    n694 = case shown="True" w888 {
      frame False {
        n695 = local write "Rd"(TRUE ("Boolean 7")) -> ()
      }
      frame True {
        n696 = flat-sequence {
          tunnel: [w928] -> w896
          tunnel: [w915] -> w894
          tunnel: [w925] -> w890
          tunnel: w896 -> [w937]
          tunnel: [w937] -> w895
          tunnel: w894 -> [w936]
          tunnel: [w936] -> w893
          tunnel: [w934] -> w892
          tunnel: [w933] -> w891
          tunnel: w890 -> [w933]
          tunnel: w895 -> [w939]
          tunnel: w893 -> [w940]
          tunnel: w892 -> [_]
          tunnel: w891 -> [w938]
          frame #0 {
            n697 = case shown="True" "Rd" {
              frame False {
              }
              frame True {
                n698 = while {
                  tunnel: "abcdefABCDEF" ("string 2") -> [w907]
                  shift-right: [w905] -> w899
                  shift-left: "" -> [w904]
                  i -> [w914]
                  stop <- w913 stop-if-true
                  n699 = Random Number (0-1)() -> (number: 0 to 1=w908:dbl)
                  n700 = Multiply(x=w908, y=62.0) -> (x*y=w910:dbl)
                  n701 = Decrement(x="Length 2") -> (x-1=w903:i16)
                  n702 = To Word Integer(number=w910) -> (16bit integer=w911:i16)
                  n703 = String Subset(string=w907, offset (0)=w911, length (rest)=1 ("length (rest)")) -> (substring=w906:string)
                  n704 = Greater Or Equal?(x=w914, y=w903) -> (x >= y?=w913:bool)
                  n705 = Concatenate Strings(w906, w904) -> (w905:string)
                }
                "String 10" <- w899
                n706 = local write "Rd"(FALSE ("Boolean 7")) -> ()
              }
            }
          }
          frame #1 {
            w926 = "_resized.jpg" ("command line")
            (unwired) ".jpg -resize 320x240 " ("string")
            (unwired) "Choose an Image File" ("prompt")
            # "-resize 1798x425"
            n707 = local read "Image Path"() -> (w920:path)
            n708 = Strip Path(path=w920) -> (stripped path=w915:path, name=w916:string)
            n709 = Match Pattern(string=w916, regular expression=".jpg") -> (before substring=→"before substring 2":string, after substring=→"after substring":string)  [unwired: 1 in, 2 out]
            n710 = Match Pattern(string=w916, regular expression="\\") -> (before substring=w922:string)  [unwired: 1 in, 3 out]
            n711 = Match Pattern(string=w922, regular expression=".jpg") -> (before substring=w921:string)  [unwired: 1 in, 3 out]
            n712 = Concatenate Strings("cmd /c convert " ("string"), w921, ".jpg -resize 320x240  " ("command line"), w921, w926) -> (w929:string)
            n713 = call <vilib>:"System Exec.vi"("run minimized? (F)"=TRUE, "wait until completion? (T)"=TRUE, "working directory"=w915, "command line"=w929) -> ("error out"=w928:errorcluster)  [unwired: 4 in, 3 out]
            "error out 2" <- w928
            n714 = Concatenate Strings(w921, w926) -> (w925:string)
          }
          frame #2 {
            n715 = Wait (ms)(milliseconds to wait=u32 2000 ("millisecond timer value")) -> (millisecond timer value=w934:u32)
          }
          frame #3 {
            n716 = case shown="No Error" w939 {
              tunnel: w940 -> [w943 _]
              tunnel: w938 -> [w941 _]
              frame No Error {
                (unwired) ".jpg" ("string")
                n717 = Path To String(path=w943) -> (string=w947:string)
                n718 = Concatenate Strings(w947, "\\" ("string"), w941) -> (w946:string)
                n719 = String To Path(string=w946) -> (path=w945:path)
                n720 = call <vilib>:"Read JPEG File.vi"("path to JPEG file"=w945) -> ("image data"=w949:T11)  [unwired: 8 in, 2 out]
                "image data" <- w949
                n721 = local write "Print 3"(FALSE ("Print 2")) -> ()
                n722 = call <vilib>:"Draw Flattened Pixmap.vi"("image data"=w949) -> ("new picture"=→"new picture":picture)  [unwired: 8 in]
              }
              frame Error {
              }
            }
          }
        }
      }
    }
    n723 = Wait (ms)(milliseconds to wait=u32 20 ("millisecond timer value")) -> ()  [unwired: 1 out]
    n724 = local read "Quit"() -> (w882:bool)
  }
  n725 = while {
    tunnel: w33 -> [_]
    tunnel: w16 -> [_]
    stop <- w980 stop-if-true
    # "New Adv Logics"
    n726 = local read "Main Tab"() -> (w959:T2)
    n727 = local read "Main Tab"() -> (w978:T2)
    n728 = local read "Sign In"() -> (w977:bool)
    n729 = case shown="\"Adv Scar\"" w959 {
      frame "HOME", Default {
        n730 = local read "LIVE FEED MIN TEMP"() -> (w1107:bool)
        n731 = local write "LIVE FEED MAX TEMP"(TRUE ("LIVE FEED MAX TEMP")) -> ()
        n732 = local read "CAMERA ROI MIN TEMP"() -> (w1105:bool)
        n733 = case shown="True" w1107 {
          selector: w1107 -> [_ w1114]
          frame False {
          }
          frame True {
            n734 = Not(x=w1114) -> (.not. x?=w1113:bool)
            n735 = local write "LIVE FEED MIN TEMP"(w1113) -> ()
            n736 = call "CAMERA LIVE FEED FGV.vi"("Enum - Menu"=CAMERA_LIVE_FEED_ENUM."CAMERA MINIMIZE") -> ()  [unwired: 9 in, 2 out]
          }
        }
        n737 = case shown="True" w1105 {
          selector: w1105 -> [_ w1111]
          frame False {
          }
          frame True {
            n738 = Not(x=w1111) -> (.not. x?=w1110:bool)
            n739 = local write "CAMERA ROI MIN TEMP"(w1110) -> ()
            n740 = call "IMAGE ANALYSIS.vi"("Enum"=POST_ANALYSIS_ENUM."MINIMIZE UI") -> ()  [unwired: 9 in, 2 out]
          }
        }
        n741 = local write "CAMERA ROI MAX TEMP"(TRUE ("CAMERA ROI MAX TEMP")) -> ()
      }
      frame "Test Setup" {
        n742 = local read "LIVE FEED MIN TEMP"() -> (w1117:bool)
        n743 = local read "CAMERA ROI MIN TEMP"() -> (w1115:bool)
        n744 = local write "LIVE FEED MAX TEMP"(TRUE ("LIVE FEED MAX TEMP")) -> ()
        n745 = case shown="True" w1117 {
          selector: w1117 -> [_ w1124]
          frame False {
          }
          frame True {
            n746 = Not(x=w1124) -> (.not. x?=w1123:bool)
            n747 = local write "LIVE FEED MIN TEMP"(w1123) -> ()
            n748 = call "CAMERA LIVE FEED FGV.vi"("Enum - Menu"=CAMERA_LIVE_FEED_ENUM."CAMERA MINIMIZE") -> ()  [unwired: 9 in, 2 out]
          }
        }
        n749 = case shown="True" w1115 {
          selector: w1115 -> [_ w1121]
          frame False {
          }
          frame True {
            n750 = Not(x=w1121) -> (.not. x?=w1120:bool)
            n751 = local write "CAMERA ROI MIN TEMP"(w1120) -> ()
            n752 = call "IMAGE ANALYSIS.vi"("Enum"=POST_ANALYSIS_ENUM."MINIMIZE UI") -> ()  [unwired: 9 in, 2 out]
          }
        }
        n753 = local write "CAMERA ROI MAX TEMP"(TRUE ("CAMERA ROI MAX TEMP")) -> ()
      }
      frame "Acquire" {
        n754 = local read "LIVE FEED MIN TEMP"() -> (w1127:bool)
        n755 = local write "LIVE FEED MAX TEMP"(TRUE ("LIVE FEED MAX TEMP")) -> ()
        n756 = local read "CAMERA ROI MIN TEMP"() -> (w1125:bool)
        n757 = case shown="True" w1127 {
          selector: w1127 -> [_ w1134]
          frame False {
          }
          frame True {
            n758 = Not(x=w1134) -> (.not. x?=w1133:bool)
            n759 = local write "LIVE FEED MIN TEMP"(w1133) -> ()
            n760 = call "CAMERA LIVE FEED FGV.vi"("Enum - Menu"=CAMERA_LIVE_FEED_ENUM."CAMERA MINIMIZE") -> ()  [unwired: 9 in, 2 out]
          }
        }
        n761 = case shown="True" w1125 {
          selector: w1125 -> [_ w1131]
          frame False {
          }
          frame True {
            n762 = Not(x=w1131) -> (.not. x?=w1130:bool)
            n763 = local write "CAMERA ROI MIN TEMP"(w1130) -> ()
            n764 = call "IMAGE ANALYSIS.vi"("Enum"=POST_ANALYSIS_ENUM."MINIMIZE UI") -> ()  [unwired: 9 in, 2 out]
          }
        }
        n765 = local write "CAMERA ROI MAX TEMP"(TRUE ("CAMERA ROI MAX TEMP")) -> ()
      }
      frame "Adv Scar" {
        n766 = local read "CAMERA ROI MIN TEMP"() -> (w1135:bool)
        n767 = case shown="True" "LIVE FEED MAX TEMP" {
          selector: "LIVE FEED MAX TEMP" -> [_ w1156]
          frame False {
          }
          frame True {
            n768 = Not(x=w1156) -> (.not. x?=w1155:bool)
            n769 = local write "LIVE FEED MAX TEMP"(w1155) -> ()
            n770 = call "CAMERA LIVE FEED FGV.vi"("Enum - Menu"=CAMERA_LIVE_FEED_ENUM."CAMERA RESTORE") -> ("error out"=w1146:errorcluster)  [unwired: 9 in, 1 out]
            n771 = Type Cast(type=30, x=0) -> (*(type *) &x=w1150:i32)
            n772 = Add(x=w1150, y=48) -> (x+y=w1151:i32)
            n773 = call "CAMERA LIVE FEED FGV.vi"("Enum - Menu"=CAMERA_LIVE_FEED_ENUM."CAMERA MODE SET", "error in (no error)"=w1146, "CAMERA MODE"=w1151) -> ("error out"=w1143:errorcluster)  [unwired: 7 in, 1 out]
            n774 = call "CAMERA LIVE FEED FGV.vi"("Enum - Menu"=CAMERA_LIVE_FEED_ENUM."CAMERA GRAY", "error in (no error)"=w1143) -> ("error out"=w1142:errorcluster)  [unwired: 8 in, 1 out]
            n775 = call "LIST FILE NAMES.vi"("error in (no error)"=w1142) -> ("error out"=w1152:errorcluster, "filenames"=w1153:string[])  [unwired: 9 in]
            n776 = property on="FILE 3" class="CmbBox"(error in=w1152, "Strings[]"=w1153) -> ()  [unwired: 1 in, 2 out]
          }
        }
        n777 = case shown="True" w1135 {
          selector: w1135 -> [_ w1141]
          frame False {
          }
          frame True {
            n778 = Not(x=w1141) -> (.not. x?=w1140:bool)
            n779 = local write "CAMERA ROI MIN TEMP"(w1140) -> ()
            n780 = call "IMAGE ANALYSIS.vi"("Enum"=POST_ANALYSIS_ENUM."MINIMIZE UI") -> ()  [unwired: 9 in, 2 out]
          }
        }
        n781 = local write "CAMERA ROI MAX TEMP"(TRUE ("CAMERA ROI MAX TEMP")) -> ()
        "LIVE FEED MIN TEMP" <- TRUE ("LIVE FEED MIN TEMP")
      }
      frame "Adv Scar Report" {
        n782 = local read "CAMERA ROI MAX TEMP"() -> (w1157:bool)
        n783 = local read "LIVE FEED MIN TEMP"() -> (w1159:bool)
        n784 = local write "LIVE FEED MAX TEMP"(TRUE ("LIVE FEED MAX TEMP")) -> ()
        n785 = case shown="True" w1159 {
          selector: w1159 -> [_ w1168]
          frame False {
          }
          frame True {
            n786 = Not(x=w1168) -> (.not. x?=w1167:bool)
            n787 = local write "LIVE FEED MIN TEMP"(w1167) -> ()
            n788 = call "CAMERA LIVE FEED FGV.vi"("Enum - Menu"=CAMERA_LIVE_FEED_ENUM."CAMERA MINIMIZE") -> ()  [unwired: 9 in, 2 out]
          }
        }
        n789 = case shown="True" w1157 {
          selector: w1157 -> [_ w1165]
          frame False {
          }
          frame True {
            n790 = Not(x=w1165) -> (.not. x?=w1163:bool)
            n791 = local write "CAMERA ROI MAX TEMP"(w1163) -> ()
            n792 = call "IMAGE ANALYSIS.vi"("Enum"=POST_ANALYSIS_ENUM."SHOW UI") -> ("error out"=w1162:errorcluster)  [unwired: 9 in, 1 out]
            n793 = call "LIST FILE NAMES.vi"("error in (no error)"=w1162) -> ("filenames"=w1161:string[])  [unwired: 9 in, 1 out]
            n794 = property on="Test File List :" class="CmbBox"("Strings[]"=w1161) -> ()  [unwired: 2 in, 2 out]
          }
        }
        n795 = local write "CAMERA ROI MIN TEMP"(TRUE ("CAMERA ROI MIN TEMP")) -> ()
      }
      frame "Compare Files" {
        n796 = local read "LIVE FEED MIN TEMP"() -> (w1171:bool)
        n797 = local write "LIVE FEED MAX TEMP"(TRUE ("LIVE FEED MAX TEMP")) -> ()
        n798 = local read "CAMERA ROI MIN TEMP"() -> (w1169:bool)
        n799 = case shown="True" w1171 {
          selector: w1171 -> [_ w1178]
          frame False {
          }
          frame True {
            n800 = Not(x=w1178) -> (.not. x?=w1177:bool)
            n801 = local write "LIVE FEED MIN TEMP"(w1177) -> ()
            n802 = call "CAMERA LIVE FEED FGV.vi"("Enum - Menu"=CAMERA_LIVE_FEED_ENUM."CAMERA MINIMIZE") -> ()  [unwired: 9 in, 2 out]
          }
        }
        n803 = case shown="True" w1169 {
          selector: w1169 -> [_ w1175]
          frame False {
          }
          frame True {
            n804 = Not(x=w1175) -> (.not. x?=w1174:bool)
            n805 = local write "CAMERA ROI MIN TEMP"(w1174) -> ()
            n806 = call "IMAGE ANALYSIS.vi"("Enum"=POST_ANALYSIS_ENUM."MINIMIZE UI") -> ()  [unwired: 9 in, 2 out]
          }
        }
